vi "ClearHWSyncedImages.vi"(0 "object in":refnum<class "Hamamatsu.lvclass">, 5 "error in (no error)":errorcluster) -> (14 "object out":refnum<class "Hamamatsu.lvclass">, 19 "error out":errorcluster)   [LabVIEW 2021, in "Hamamatsu.lvclass"]
uses:
  Hamamatsu.lvclass
  <vilib>/vision/Image Controls.llb/IMAQ Image.ctl
  Hamamatsu.lvclass/Hamamatsu.ctl
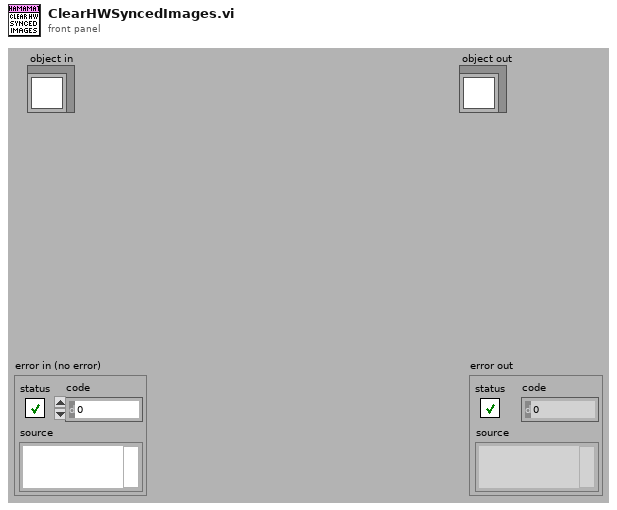
[diagram p1: front panel]
types:
  T1 = typedef "IMAQ Image.ctl" = refnum<image>
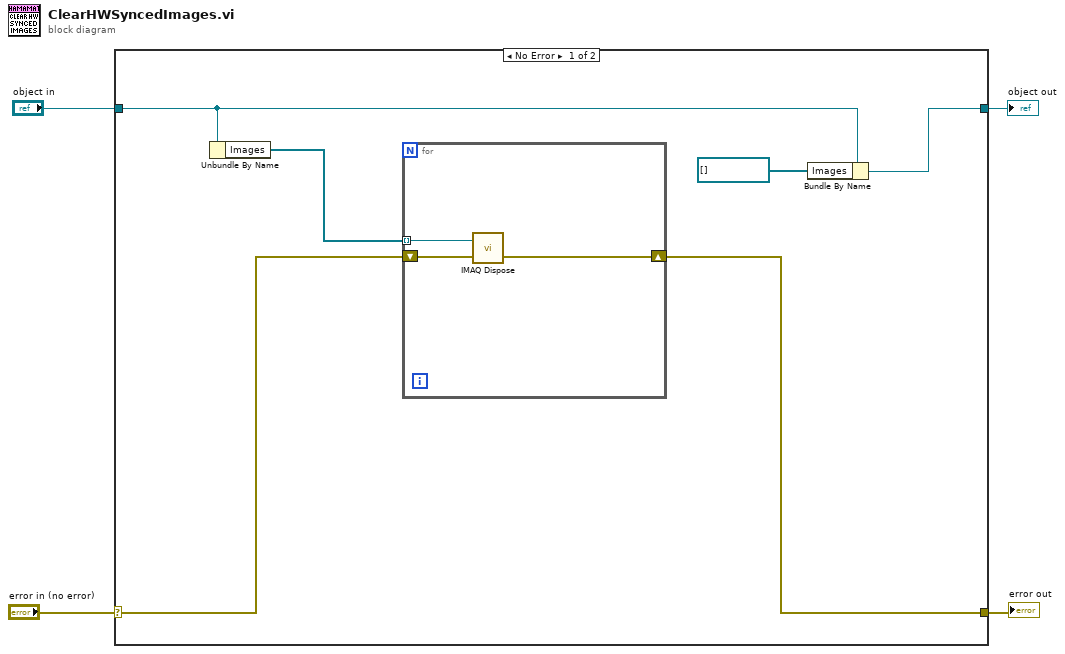
[diagram p0: block diagram]
diagram:
  n1 = case shown="No Error" "error in (no error)" {
    selector: "error in (no error)" -> [w9 w15]
    tunnel: [w8 w15] -> w3
    tunnel: [w7 w14] -> w1
    tunnel: "object in" -> [w6 w14]
    frame No Error {
      n2 = Unbundle By Name(w6) -> ("Images"=w10:T1[])
      n3 = for {
        tunnel: w10 -> [w13] mode=indexing
        shift-right: [w11] -> w8
        shift-left: w9 -> [w12]
        n4 = call "IMAQ Dispose"("Image"=w13, "error in (no error)"=w12) -> ("error out"=w11:errorcluster)  [unwired: 4 in]
      }
      n5 = Bundle By Name(cluster=w6, "Images"=T1[] [] ("HWSyncedImages")) -> (w7:refnum<class "Hamamatsu.lvclass">)
    }
    frame Error {
    }
  }
  "error out" <- w3
  "object out" <- w1
